vi "img test 5(extract court).vi"() -> ()   [LabVIEW 2009]
uses:
  <vilib>/vision/NI_Vision_Development_Module.lvlib
panel:
  out "Image 4":T1(plugin-control)
  out "Image Pixels (U8)":u8[][](array[numeric])
  out "Image 3":T1(plugin-control)
  out "Image 2":T1(plugin-control)
  in  "x+y":i32
  in  "AVI Path":path=path "C:/Users/Kokum Weeratunga/Desktop/img processing/ChongWei vs LinDan (japan open 2010).avi"
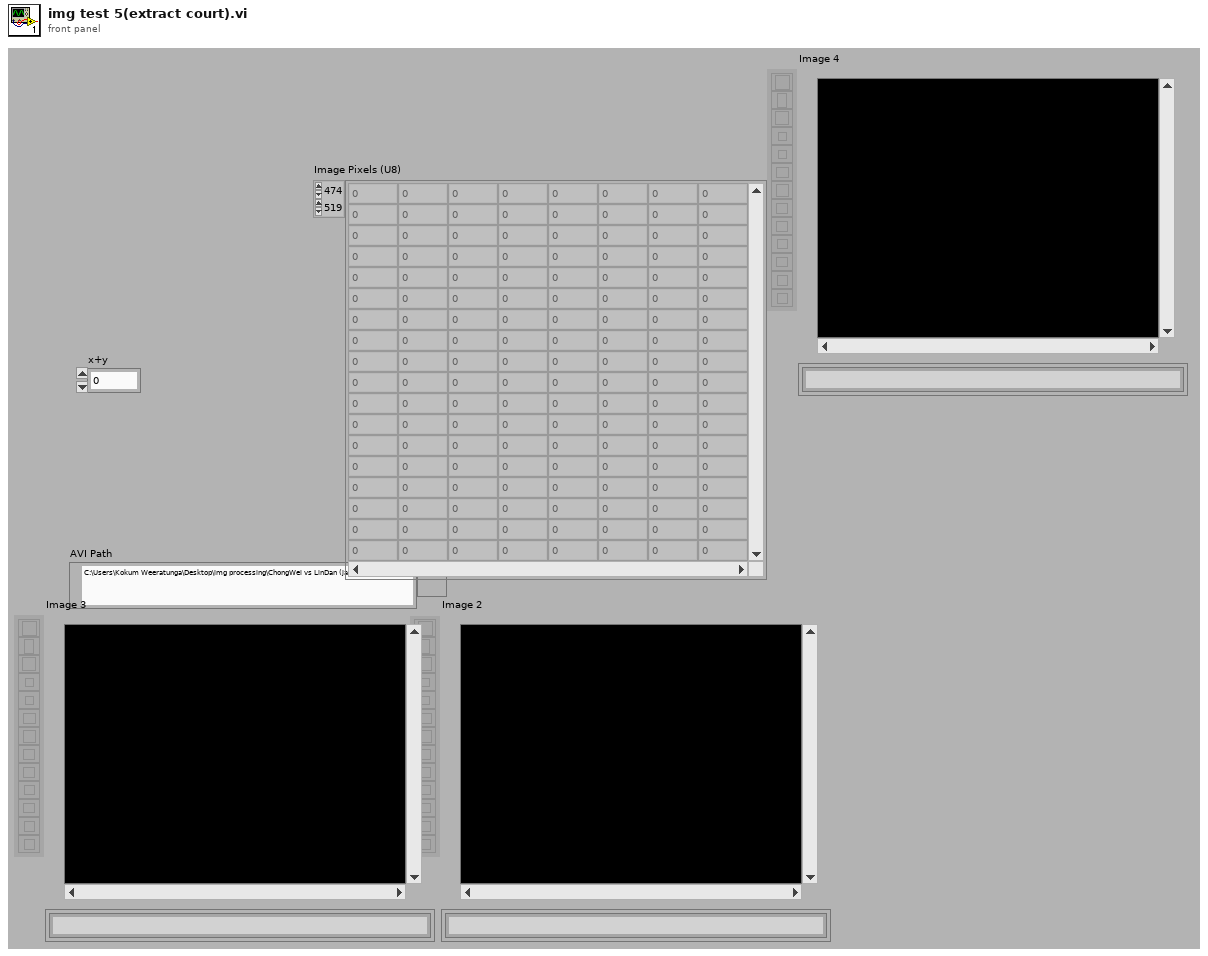
[diagram p1: front panel]
types:
  T1 = typedef "IMAQ Image.ctl" = refnum<image>
  T2 = typedef "Image Type" = u32
  T3 = enum32{"AutoM", "Close", "Dilate", "Erode", "Gradient", "Gradient in", "Gradient out", "HitMiss", "Open", "PClose", "POpen", "Thick", "Thin"}
  T4 = typedef "AviRefnum.ctl" = refnum<k1>
  T5 = cluster{"Starting Value":sgl, "Incremental Value":sgl, "Histogram":u32[]}
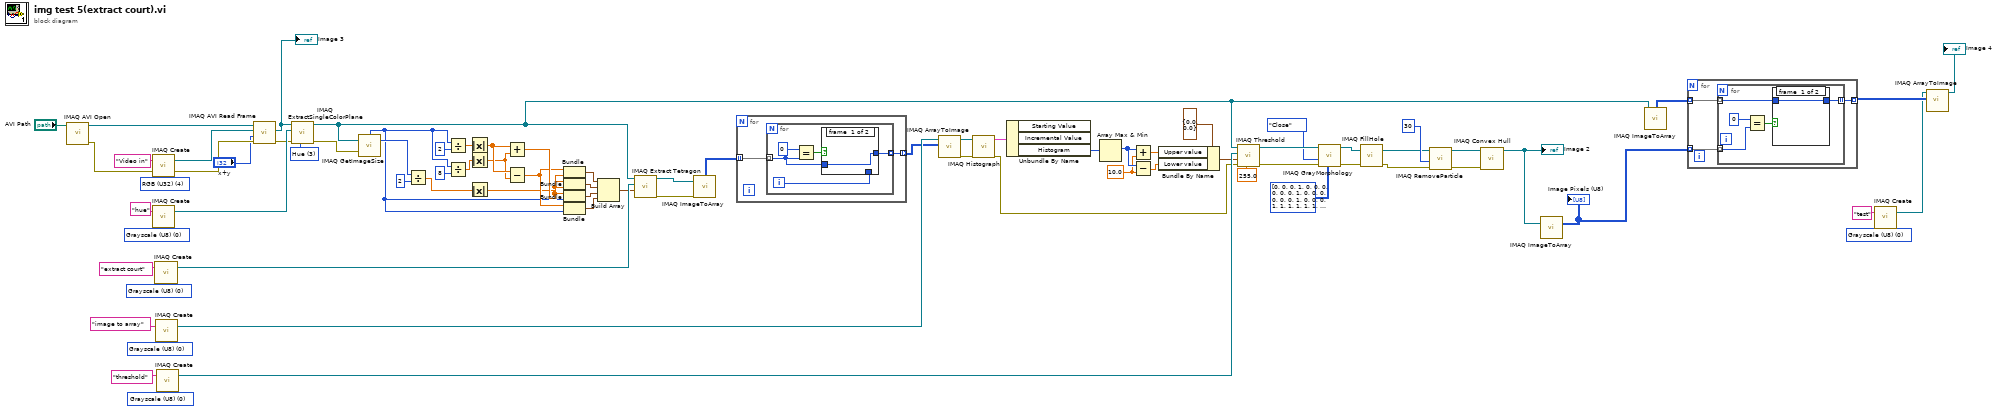
[diagram p0: block diagram]
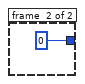
[diagram p2: hidden frame]
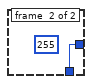
[diagram p3: hidden frame]
diagram:
  w5 = T2 0 items=["Grayscale (U8)", "Grayscale (I16)", "Grayscale (SGL)", "Complex (CSG)", "RGB (U32)", "HSL (U32)", "RGB (U64)", "Grayscale (U16)"] ("Image Type")
  w58 = 3 items=["Red", "Green", "Blue", "Hue", "Saturation", "Luminance", "Value", "Intensity"] ("Color Plane")
  w30 = sgl 10.0 ("Upper value")
  w68 = T2 0 items=["Grayscale (U8)", "Grayscale (I16)", "Grayscale (SGL)", "Complex (CSG)", "RGB (U32)", "HSL (U32)", "RGB (U64)", "Grayscale (U16)"] ("Image Type")
  w66 = T2 0 items=["Grayscale (U8)", "Grayscale (I16)", "Grayscale (SGL)", "Complex (CSG)", "RGB (U32)", "HSL (U32)", "RGB (U64)", "Grayscale (U16)"] ("Image Type")
  w70 = T2 0 items=["Grayscale (U8)", "Grayscale (I16)", "Grayscale (SGL)", "Complex (CSG)", "RGB (U32)", "HSL (U32)", "RGB (U64)", "Grayscale (U16)"] ("Image Type")
  w72 = T2 0 items=["Grayscale (U8)", "Grayscale (I16)", "Grayscale (SGL)", "Complex (CSG)", "RGB (U32)", "HSL (U32)", "RGB (U64)", "Grayscale (U16)"] ("Image Type")
  w74 = T2 4 items=["Grayscale (U8)", "Grayscale (I16)", "Grayscale (SGL)", "Complex (CSG)", "RGB (U32)", "HSL (U32)", "RGB (U64)", "Grayscale (U16)"] ("Image Type")
  n1 = call "IMAQ AVI Open"("AVI Path"="AVI Path") -> ("error out"=w60:errorcluster, "Avi Refnum"=w61:T4)  [unwired: 9 in]
  n2 = call "IMAQ Create"("Image Name"="Video in", "Image Type"=w74, "error in (no error)"=w60) -> ("New Image"=w75:T1, "error out"=w76:errorcluster)  [unwired: 2 in]
  n3 = call "IMAQ Create"("Image Name"="hue", "Image Type"=w72) -> ("New Image"=w71:T1)  [unwired: 3 in, 1 out]
  n4 = call "IMAQ Create"("Image Name"="extract court", "Image Type"=w66) -> ("New Image"=w64:T1)  [unwired: 3 in, 1 out]
  n5 = call "IMAQ Create"("Image Name"="image to array", "Image Type"=w68) -> ("New Image"=w63:T1)  [unwired: 3 in, 1 out]
  n6 = call "IMAQ Create"("Image Name"="threshold", "Image Type"=w70) -> ("New Image"=w62:T1)  [unwired: 3 in, 1 out]
  n7 = call "IMAQ AVI Read Frame"("error in (no error)"=w76, "Frame Number"="x+y", "Image"=w75, "Avi Refnum"=w61) -> ("error out"=w25:errorcluster, "Image Out"=w14:T1)  [unwired: 4 in, 2 out]
  "Image 3" <- w14
  n8 = call "IMAQ ExtractSingleColorPlane"("Color Plane"=w58, "error in (no error)"=w25, "Image Dst"=w71, "Image Src"=w14) -> ("error out"=w24:errorcluster, "Image Dst Out"=w7:T1)  [unwired: 6 in]
  n9 = call "IMAQ GetImageSize"("Image"=w7, "error in (no error)"=w24) -> ("Y Resolution"=w56:i32, "X Resolution"=w40:i32)  [unwired: 2 in, 1 out]
  n10 = Divide(x=w56, y=2) -> (x/y=w51:dbl)
  n11 = Divide(x=w40, y=2) -> (x/y=w48:dbl)
  n12 = Divide(x=w40, y=8) -> (x/y=w49:dbl)
  n13 = Absolute Value(x=w48) -> (abs(x)=w47:dbl)
  n14 = Absolute Value(x=w49) -> (abs(x)=w46:dbl)
  n15 = Absolute Value(x=w51) -> (abs(x)=w50:dbl)
  n16 = Add(x=w47, y=w46) -> (x+y=w53:dbl)
  n17 = Subtract(x=w47, y=w46) -> (x-y=w52:dbl)
  n18 = Bundle(w52, w50) -> (w45:cluster{dbl, dbl})  [unwired: 1 in]
  n19 = Bundle(w53, w50) -> (w44:cluster{dbl, dbl})  [unwired: 1 in]
  n20 = Bundle(w53, "X Resolution"=w40) -> (w43:cluster{dbl, "X Resolution":i32})  [unwired: 1 in]
  n21 = Bundle(w52, "X Resolution"=w40) -> (w42:cluster{dbl, "X Resolution":i32})  [unwired: 1 in]
  n22 = Build Array(w45, w44, w43, w42) -> (w41:cluster{dbl, "X Resolution":dbl}[])
  n23 = call-poly "IMAQ Extract Tetragon"("Tetragon"=w41, "Image Dst"=w64, "Image Src"=w7) -> ("error out"=w28:errorcluster, "Image Dst Out"=w37:T1)  [unwired: 7 in]
  n24 = call "IMAQ ImageToArray"("error in (no error)"=w28, "Image"=w37) -> ("Image Pixels (U8)"=w39:u8[][])  [unwired: 2 in, 4 out]
  n25 = for {
    tunnel: w39 -> [w80] mode=indexing
    tunnel: [w79] -> w38 mode=indexing
    n26 = for {
      tunnel: w80 -> [w82] mode=indexing
      tunnel: [w83] -> w79 mode=indexing
      i -> [w81]
      n27 = Equal?(x=u8 0, y=w82) -> (x = y?=w84:bool)
      n28 = case shown="False" w84 {
        tunnel: [w86 w87] -> w83
        tunnel: w82 -> [w86 _]
        tunnel: w81 -> [_ w87]
        frame #0 {
        }
        frame #1 {
          (unwired) u8 255 ("x")
        }
      }
    }
  }
  n29 = call "IMAQ ArrayToImage"("Image Pixels (U8)"=w38, "Image"=w63) -> ("error out"=w23:errorcluster, "Image Out"=w36:T1)  [unwired: 8 in]
  n30 = call "IMAQ Histograph"("error in (no error)"=w23, "Image"=w36) -> ("error out"=w22:errorcluster, "Histogram Graph"=w35:T5)  [unwired: 6 in, 2 out]
  n31 = Unbundle By Name(w35) -> ("Histogram"=w34:u32[])  [unwired: 2 out]
  n32 = Array Max & Min(array=w34) -> (max index (indices)=w33:i32)  [unwired: 3 out]
  n33 = Add(x=w33, y=w30) -> (x+y=w27:sgl)
  n34 = Subtract(x=w33, y=w30) -> (x-y=w26:sgl)
  n35 = Bundle By Name(cluster=cluster{"Lower value":sgl, "Upper value":sgl} {"Lower value"=0.0, "Upper value"=0.0} ("Range"), "Upper value"=w27, "Lower value"=w26) -> (w32:cluster{"Lower value":sgl, "Upper value":sgl})
  n36 = call "IMAQ Threshold"("Replace Value"=sgl 255.0, "error in (no error)"=w22, "Range"=w32, "Image Dst"=w62, "Image Src"=w7) -> ("error out"=w12:errorcluster, "Image Dst Out"=w21:T1)  [unwired: 5 in]
  n37 = call "IMAQ GrayMorphology"("Structuring Element"=i32[][] [[0, 0, 0, 1, 0, 0, 0], [0, 0, 0, 1, 0, 0, 0], [0, 0, 0, 1, 0, 0, 0], [1, 1, 1, 1, 1, 1, 1], [0, 0, 0, 1, 0, 0, 0], [0, 0, 0, 1, 0, 0, 0], [0, 0, 0, 1, 0, 0, 0]], "error in (no error)"=w12, "Operation"=T3."Close", "Image Src"=w21) -> ("error out"=w17:errorcluster, "Image Dst Out"=w18:T1)  [unwired: 6 in]
  n38 = call "IMAQ FillHole"("error in (no error)"=w17, "Image Src"=w18) -> ("error out"=w11:errorcluster, "Image Dst Out"=w15:T1)  [unwired: 4 in]
  n39 = call "IMAQ RemoveParticle"("error in (no error)"=w11, "Number of Erosion"=30, "Image Src"=w15) -> ("error out"=w10:errorcluster, "Image Dst Out"=w13:T1)  [unwired: 7 in]
  n40 = call "IMAQ Convex Hull"("error in (no error)"=w10, "Image Src"=w13) -> ("Image Dst Out"=w9:T1)  [unwired: 8 in, 1 out]
  "Image 2" <- w9
  n41 = call "IMAQ ImageToArray"("Image"=w9) -> ("Image Pixels (U8)"=w6:u8[][])  [unwired: 3 in, 4 out]
  "Image Pixels (U8)" <- w6
  n42 = call "IMAQ ImageToArray"("Image"=w7) -> ("Image Pixels (U8)"=w8:u8[][])  [unwired: 3 in, 4 out]
  n43 = for {
    tunnel: w8 -> [w90] mode=indexing
    tunnel: [w89] -> w3 mode=indexing
    tunnel: w6 -> [w88] mode=indexing
    n44 = for {
      tunnel: w90 -> [w92] mode=indexing
      tunnel: [w93] -> w89 mode=indexing
      tunnel: w88 -> [w91] mode=indexing
      n45 = Equal?(x=u8 0, y=w91) -> (x = y?=w94:bool)
      n46 = case shown="True" w94 {
        tunnel: [w96 u8 0 ("x")] -> w93
        tunnel: w92 -> [w96 _]
        frame #0 {
        }
        frame #1 {
        }
      }
    }
  }
  n47 = call "IMAQ Create"("Image Name"="test", "Image Type"=w5) -> ("New Image"=w2:T1)  [unwired: 3 in, 1 out]
  n48 = call "IMAQ ArrayToImage"("Image Pixels (U8)"=w3, "Image"=w2) -> ("Image Out"=→"Image 4":T1)  [unwired: 8 in, 1 out]
